vi "Scan Setup.vi"(8 "error in (no error)":errorcluster, 11 "LCD Reader in":refnum<class "LCD Reader.lvclass">) -> (0 "error out":errorcluster, 3 "LCD Reader out":refnum<class "LCD Reader.lvclass">)   [LabVIEW 2017, in "LCD Reader.lvclass"]
doc: "(Dynamic) Send commands to configure the instrument based on the class member data."
uses:
  LCD Reader.lvclass
  LCD Reader.lvclass/LCD Reader.ctl
  Reader/Reader.lvclass
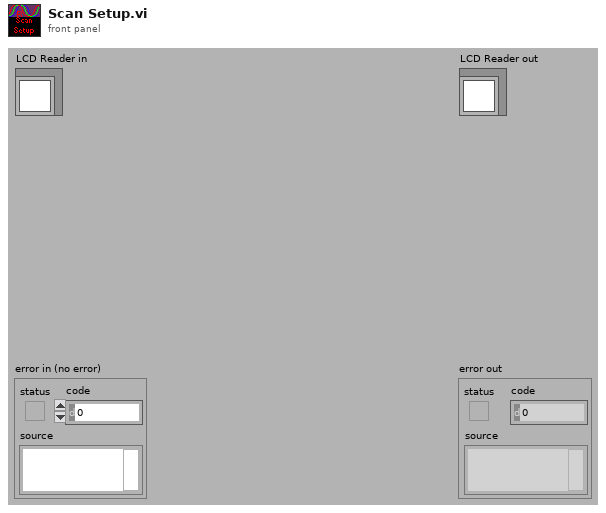
[diagram p1: front panel]
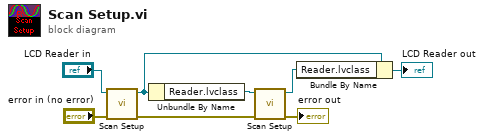
[diagram p0: block diagram]
diagram:
  n1 = call-parent "Scan Setup.vi"("error in (no error)"="error in (no error)", "Reader in"="LCD Reader in") -> ("error out"=w2:errorcluster, "Reader out"=w6:refnum<class "LCD Reader.lvclass">)  [unwired: 8 out]
  n2 = Unbundle By Name(w6) -> ("Reader.lvclass"=w5:refnum<class "Reader.lvclass">)
  n3 = call-dynamic "Scan Setup.vi"("error in (no error)"=w2, "Reader in"=w5) -> ("error out"=→"error out":errorcluster, "Reader out"=w3:refnum<class "Reader.lvclass">)  [unwired: 8 out]
  n4 = Bundle By Name(cluster=w6, "Reader.lvclass"=w3) -> (→"LCD Reader out":refnum<class "LCD Reader.lvclass">)
